vi "Main RT.vi"() -> ()   [LabVIEW 2020]
uses:
  Control/State - Main RT.ctl
  Control/Config File Section List.ctl
panel:
  out "error out":errorcluster
  in  "error in (no error)":errorcluster
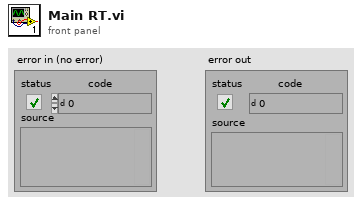
[diagram p1: front panel]
types:
  T1 = typedef "State - Main RT.ctl" = enum16{"Init module", "Register for event", "Init FGV and eFGV", "Read config file", "Idle", "Process", "Unregister user event", "Close module"}
  T2 = typedef "Config File Section List.ctl" = enum16{"RasPi Setting", "MQTT Server Setting", "MQTT Client Setting"}
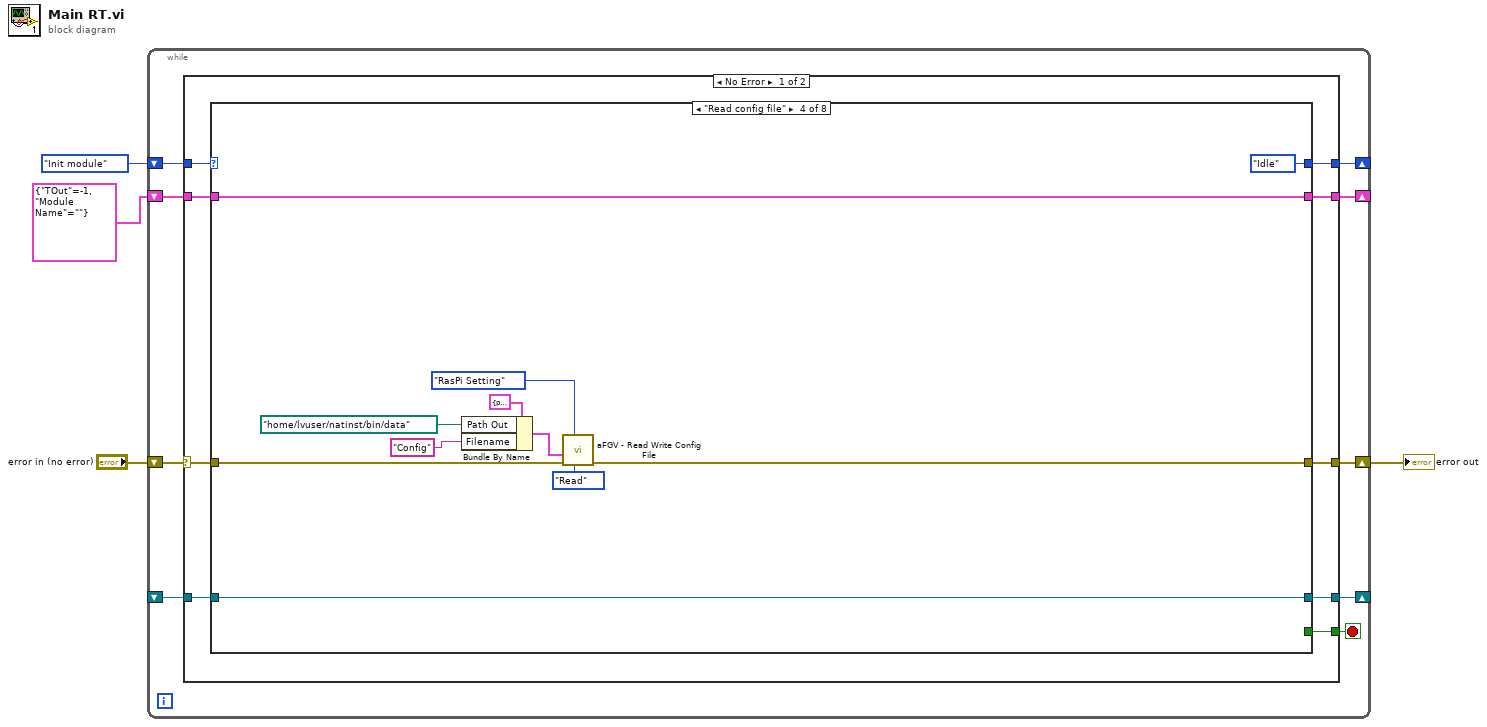
[diagram p0: block diagram]
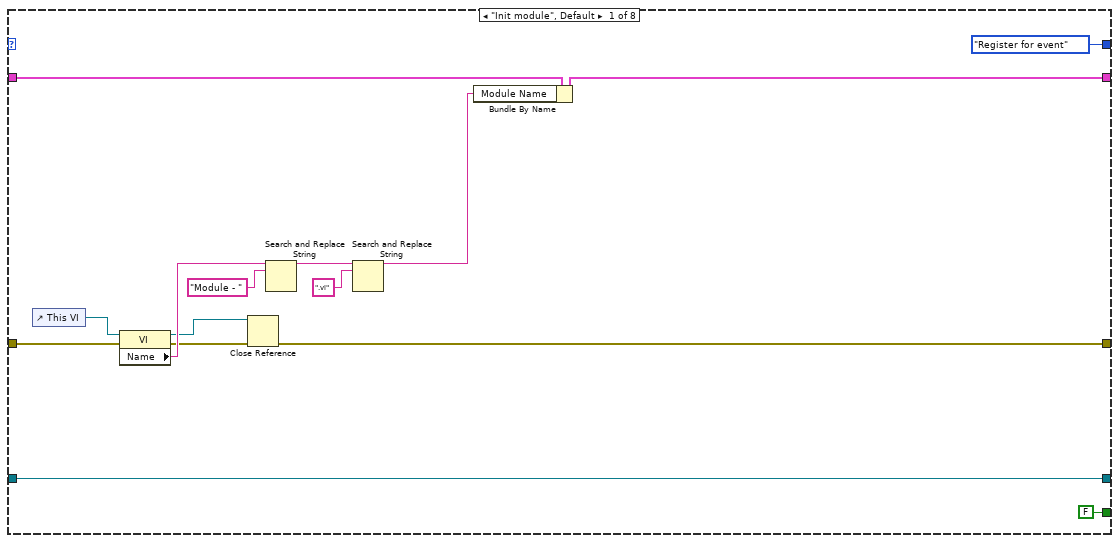
[diagram p2: hidden frame]
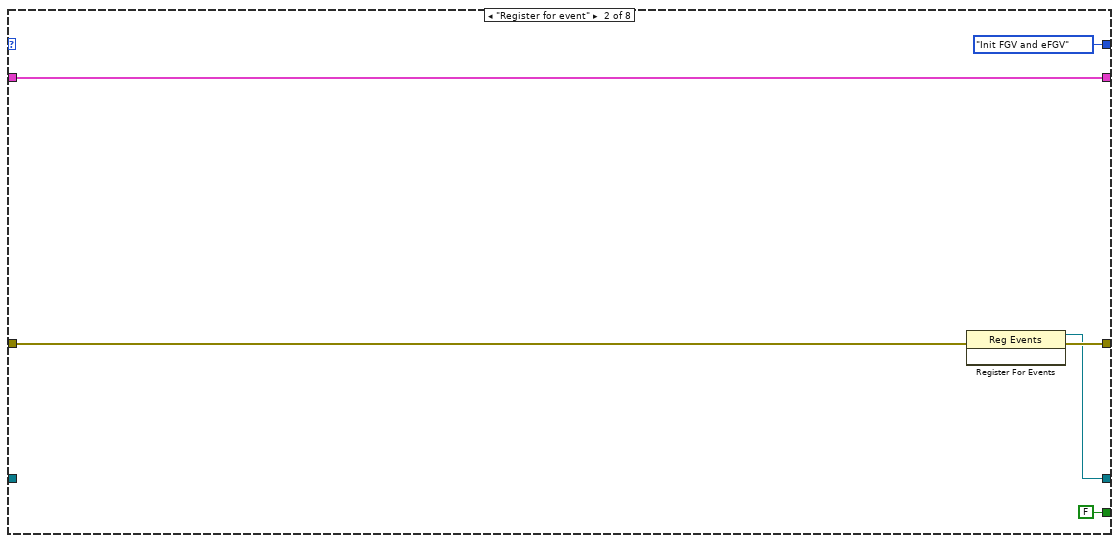
[diagram p3: hidden frame]
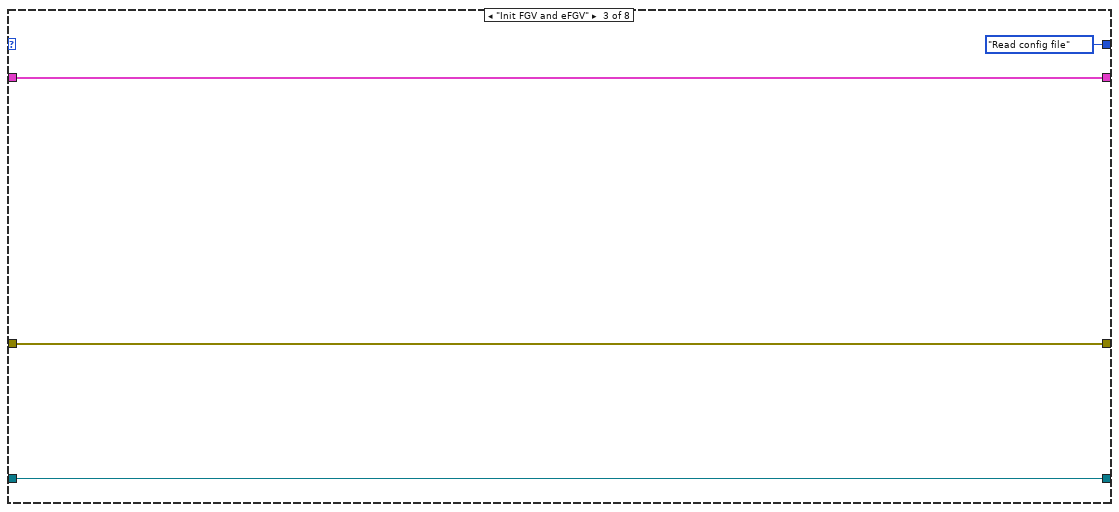
[diagram p4: hidden frame]
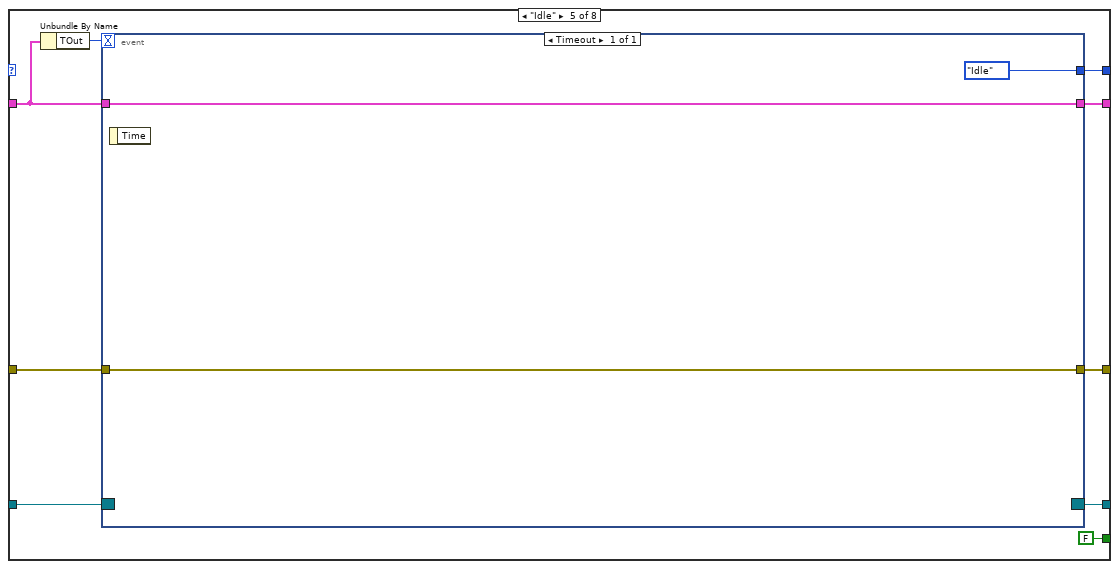
[diagram p5: hidden frame]
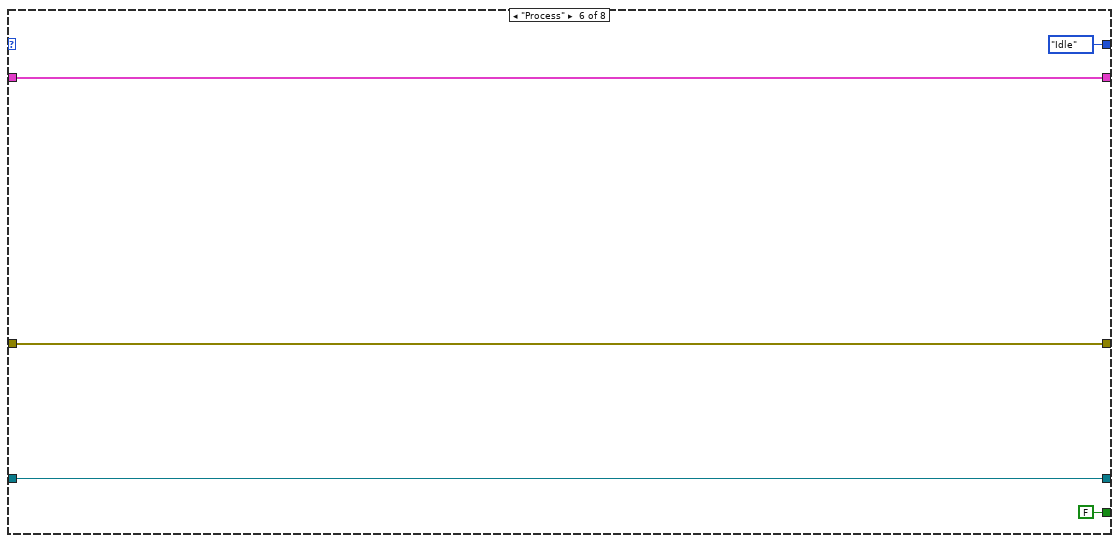
[diagram p6: hidden frame]
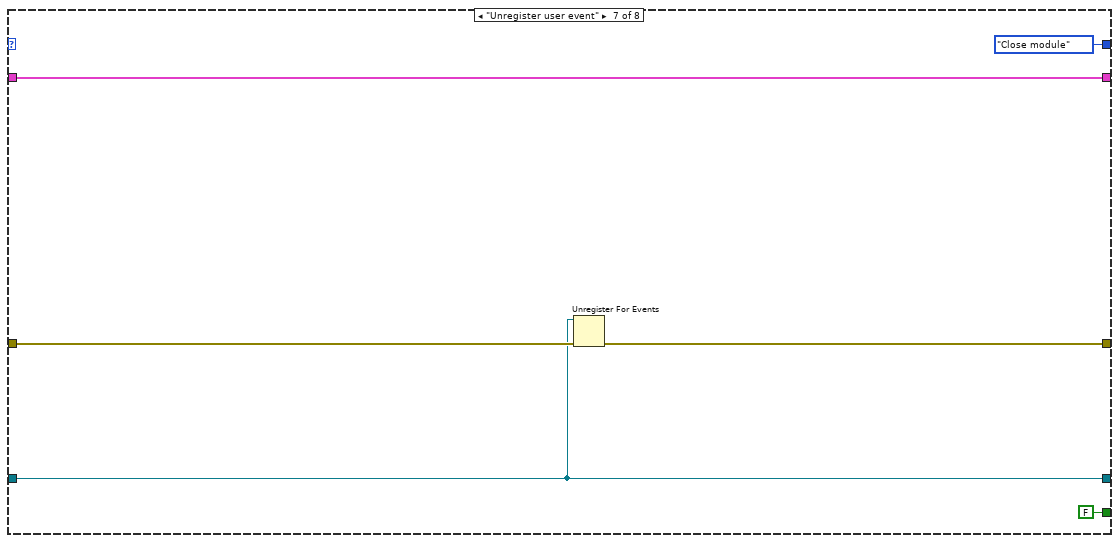
[diagram p7: hidden frame]
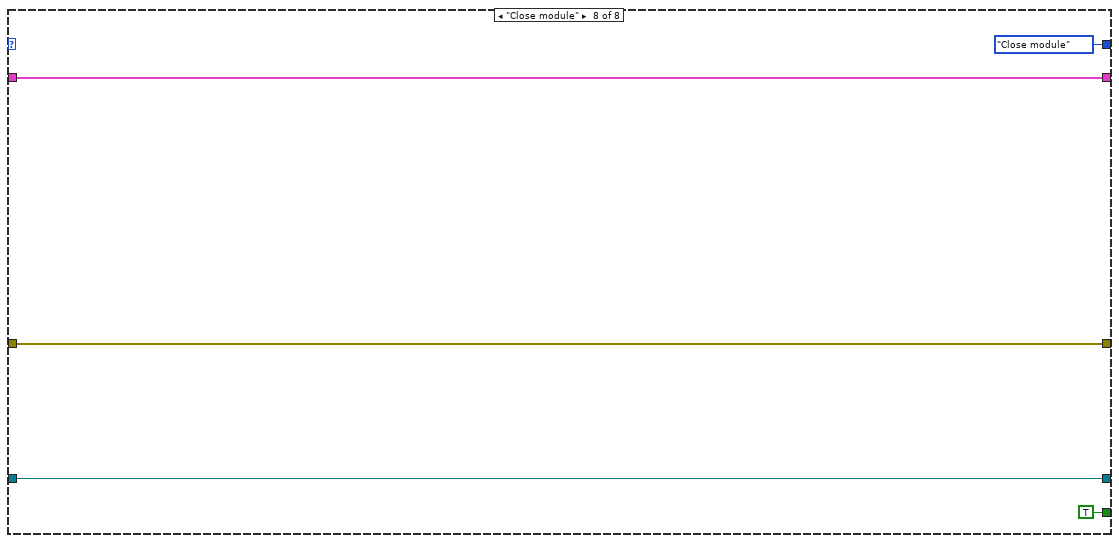
[diagram p8: hidden frame]
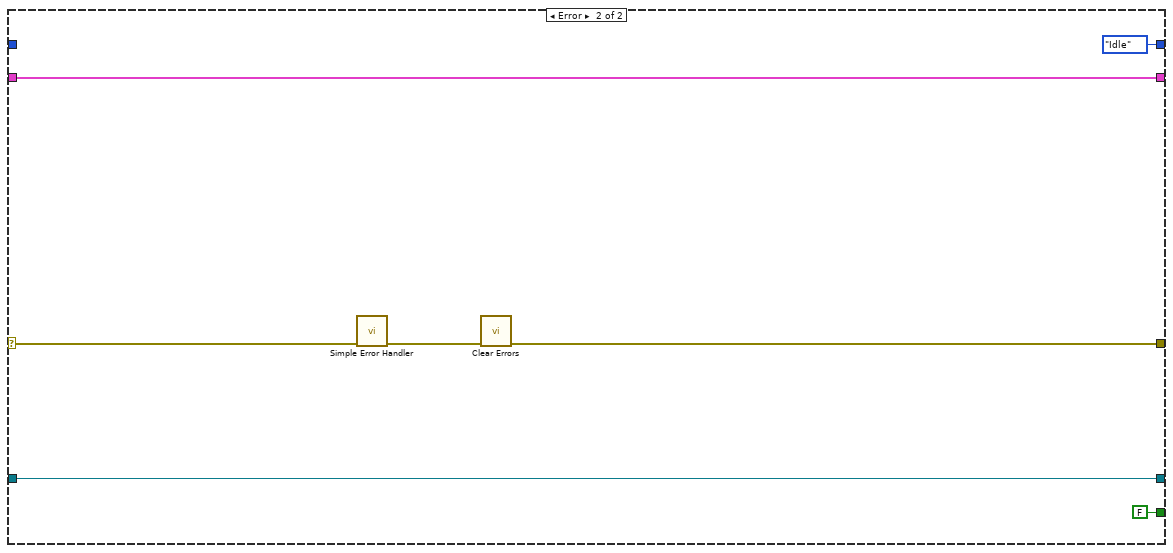
[diagram p9: hidden frame]
diagram:
  n1 = while {
    shift-right: [w9] -> w3
    shift-left: "error in (no error)" -> [w13]
    shift-right: [w5] -> _
    shift-left: State_-_Main_RT."Init module" -> [w11]
    shift-right: [w8] -> _
    shift-left: cluster{"TOut":i32, "Module Name":string} {"TOut"=-1, "Module Name"=""} -> [w10]
    shift-right: [w7] -> _
    shift-left: _ -> [w6]
    stop <- w12 stop-if-true
    n2 = case shown="No Error" w13 {
      selector: w13 -> [w22 w91]
      tunnel: [w21 FALSE] -> w12
      tunnel: w11 -> [w20 _]
      tunnel: w10 -> [w19 w88]
      tunnel: [w18 w89] -> w9
      tunnel: [w17 w88] -> w8
      tunnel: [w16 w92] -> w7
      tunnel: w6 -> [w15 w92]
      tunnel: [w14 State_-_Main_RT."Idle"] -> w5
      frame No Error {
        n3 = case shown="\"Read config file\"" w20 {
          tunnel: w22 -> [w27 w41 w47 w55 w65 w75 w80 w86]
          tunnel: [FALSE FALSE _ _ FALSE FALSE FALSE TRUE] -> w21
          tunnel: w19 -> [w36 w39 w46 w58 w62 w74 w81 w85]
          tunnel: [w26 w42 w47 w54 w64 w75 w79 w86] -> w18
          tunnel: [w25 w39 w46 w58 w61 w74 w81 w85] -> w17
          tunnel: [w35 w40 w45 w57 w66 w73 w78 w84] -> w16
          tunnel: w15 -> [w35 _ w45 w57 w67 w73 w78 w84]
          tunnel: [State_-_Main_RT."Register for event" State_-_Main_RT."Init FGV and eFGV" State_-_Main_RT."Read config file" State_-_Main_RT."Idle" w59 State_-_Main_RT."Idle" State_-_Main_RT."Close module" State_-_Main_RT."Close module"] -> w14
          frame "Init module", Default {
            n4 = control-ref of="This VI"() -> (w34:refnum<vi>)
            n5 = property class="VI"(reference=w34, error in=w27) -> (reference out=w28:refnum<vi>, error out=w29:errorcluster, "Name"=w33:string)
            n6 = Close Reference(reference=w28, error in (no error)=w29) -> (error out=w26:errorcluster)
            n7 = Search and Replace String(input string=w33, search string="Module - ") -> (result string=w30:string)  [unwired: 6 in, 3 out]
            n8 = Search and Replace String(input string=w30, search string=".vi") -> (result string=w24:string)  [unwired: 6 in, 3 out]
            n9 = Bundle By Name(cluster=w36, "Module Name"=w24) -> (w25:cluster{"TOut":i32, "Module Name":string})
          }
          frame "Register for event" {
            n10 = register-events(error in=w41) -> (reference out=w40:refnum<event-registration>, error out=w42:errorcluster)  [unwired: 2 in]
          }
          frame "Init FGV and eFGV" {
          }
          frame "Read config file" {
            n11 = Bundle By Name(cluster=cluster{"Path Out":path, "Filename":string} {"Path Out"=path "", "Filename"=""} ("Path File"), "Path Out"=path "/home/lvuser/natinst/bin/data", "Filename"="Config") -> (w51:cluster{"Path Out":path, "Filename":string})
            n12 = call "aFGV - Read Write Config File.vi"("State"=enum16{"Read", "Write", "Delete"}."Read", "Section"=Config_File_Section_List."RasPi Setting", "Error In"=w55, "Path File"=w51) -> ("Error Out"=w54:errorcluster)  [unwired: 5 in, 2 out]
          }
          frame "Idle" {
            n13 = Unbundle By Name(w62) -> ("TOut"=w63:i32)
            n14 = event shown="[0] Timeout" {
              selector: w67 -> [_]
              dyn-events: [_] -> w66
              timeout: w63 -> [_]
              tunnel: w65 -> [w70]
              tunnel: [w70] -> w64
              tunnel: w62 -> [w69]
              tunnel: [w69] -> w61
              tunnel: [State_-_Main_RT."Idle"] -> w59
              event Timeout {
                n15 = event-data() -> ()  [unwired: 1 in, 1 out]
              }
            }
          }
          frame "Process" {
          }
          frame "Unregister user event" {
            n16 = Unregister For Events(event registration refnum=w78, error in=w80) -> (error out=w79:errorcluster)
          }
          frame "Close module" {
          }
        }
      }
      frame Error {
        n17 = call <vilib>:"Simple Error Handler.vi"("error in (no error)"=w91) -> ("error out"=w90:errorcluster)  [unwired: 4 in, 4 out]
        n18 = call <vilib>:"Clear Errors.vi"("error in (no error)"=w90) -> ("error out"=w89:errorcluster)  [unwired: 5 in, 1 out]
      }
    }
  }
  "error out" <- w3
